vi "BRig_Host_dataRunState_idx_dataTS.vi"() -> (2 "output_idx_dataTS":i32)   [LabVIEW 2014]
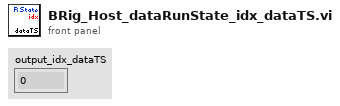
[diagram p1: front panel]
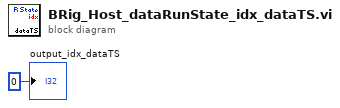
[diagram p0: block diagram]
diagram:
  "output_idx_dataTS" <- 0 ("output_idx_dataTS")
